vi "USB Scan Device.vi"(11 "pDevHandle":i32[](array[numeric])=[0, 0, 0, 0, 0, 0, 0, 0, 0, 0, 0, 0, 0, 0, 0, 0, 0, 0, 0, 0]) -> (2 "function return":i32, 3 "pDevHandle out":i32[](array[numeric]))   [LabVIEW 2010, in "usb_device.lvlib"]
doc: "int WINAPI USB_ScanDevice(int *pDevHandle);"
uses:
  usb_device.lvlib
  USB2XXX.dll
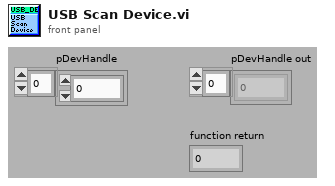
[diagram p1: front panel]
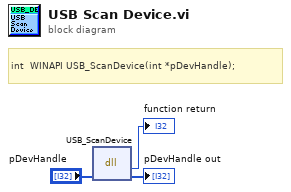
[diagram p0: block diagram]
diagram:
  # "int  WINAPI USB_ScanDevice(int *pDevHandle);"
  n1 = dll-call lib="G:/OtherWork/USB2XXX_Example/trunk/Labview/PublicFiles/USB2XXX.*" fn="USB_ScanDevice"("pDevHandle"="pDevHandle") -> (→"function return":i32, "pDevHandle"=→"pDevHandle out":i32[])  [unwired: 3 in, 2 out]
